vi "Register Abortable.vi"(8 "error in (no error)":errorcluster, 9 "Task ID":string, 10 "EnQr":refnum<class "Message Enqueuer.lvclass">, 11 "AbortManagerAPI in":refnum<class "AbortManagerAPI.lvclass">) -> (0 "error out":errorcluster, 3 "AbortManagerAPI out":refnum<class "AbortManagerAPI.lvclass">)   [LabVIEW 2020, in "Volatus.lvlib" / "AbortManagerAPI.lvclass"]
uses:
  AbortManagerAPI.lvclass
  <vilib>/ActorFramework/Message Enqueuer/Message Enqueuer.lvclass
  AbortManagerAPI.lvclass/AbortManagerAPI.ctl
  AbortManager Messages/Register Abortable Msg/Register Abortable Msg.lvclass
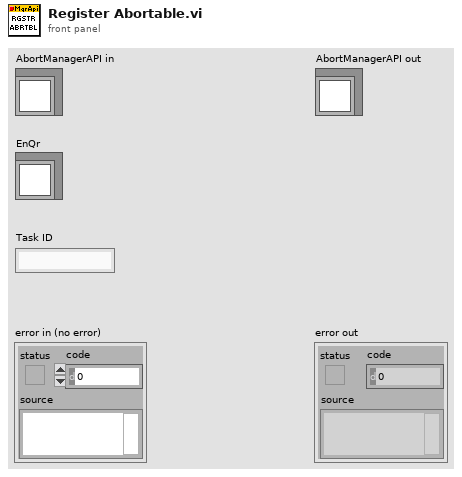
[diagram p1: front panel]
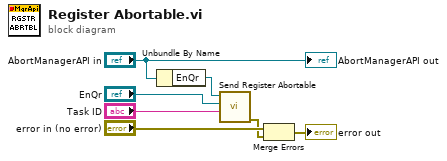
[diagram p0: block diagram]
diagram:
  n1 = Unbundle By Name("AbortManagerAPI in") -> ("EnQr"=w3:refnum<class "Message Enqueuer.lvclass">)
  n2 = call "Send Register Abortable.vi"("Task ID"="Task ID", "EnQr"="EnQr", "Message Enqueuer"=w3) -> ("error out"=w1:errorcluster)  [unwired: 7 in, 1 out]
  n3 = Merge Errors("error in (no error)", w1) -> (→"error out":errorcluster)
  "AbortManagerAPI out" <- "AbortManagerAPI in"
